vi "Modulacion FM.vi"() -> ()   [LabVIEW 2014]
doc: "This example demonstrates how to simulate a Frequency Modulation (FM) using the signal generation functions. This VI also presents the Power Spectrum of the FM signal."
uses:
  <vilib>/measure/maspectr.llb/FFT Power Spectrum and PSD for 1 Chan.vi
  <vilib>/measure/NI_MABase.lvlib
  <vilib>/measure/NI_MAPro.lvlib
panel:
  in  "Informacion de muestreo":cluster{"Fs":dbl, "#s":dbl}={"Fs"=4000000.0, "#s"=200.0} {"#s" format="%.2p"}
  in  "Frecuencia de Portadora":dbl(knob)=476774.62691567314 min=86453.20197044335 scale=62781.48791441017..1000000.0 scale format="%#_6p"
  in  "Desviacion de frecuencia\n(Maxima separacion entre\nla frecuencia modulada y\nla portadora).":dbl(slide)=35983.91523891873 scale=1.0..476774.62691567314 scale format="%#_6p"
  in  "Forma del del mensaje":T1(ring)=enum."Square Wave"
  in  "Frecuencia de mensaje":dbl(knob)=62781.48791441017 scale=1.0..100000.0 scale format="%#_6p"
  in  "Tab Control":T2(tab)=enum."Señal modulada y repsuesta en frecuencia"
  out "Mensaje":waveform(dbl)(graph)={"t0"=timestamp(0 s since 1904-01-01), "dt"=2.5e-07, "Y"=[1.0, 1.0, 1.0, 1.0, 1.0, 1.0, 1.0, 1.0, 1.0, 1.0, 1.0, 1.0, 1.0, 1.0, 1.0, 1.0, 1.0, 1.0, 1.0, 1.0, 1.0, 1.0, 1.0, 1.0, 1.0, 1.0, 1.0, 1.0, 1.0, 1.0, 1.0, 1.0, -1.0, -1.0, -1.0, -1.0, -1.0, -1.0, -1.0, -1.0, -1.0, -1.0, -1.0, -1.0, -1.0, -1.0, -1.0, -1.0, -1.0, -1.0, -1.0, -1.0, -1.0, -1.0, -1.0, -1.0, -1.0, -1.0, -1.0, -1.0, -1.0, -1.0, -1.0, -1.0, 1.0, 1.0, 1.0, 1.0, 1.0, 1.0, 1.0, 1.0, 1.0, 1.0, 1.0, 1.0, 1.0, 1.0, 1.0, 1.0, 1.0, 1.0, 1.0, 1.0, 1.0, 1.0, 1.0, 1.0, 1.0, 1.0, 1.0, 1.0, 1.0, 1.0, 1.0, 1.0, -1.0, -1.0, -1.0, -1.0, -1.0, -1.0, -1.0, -1.0, -1.0, -1.0, -1.0, -1.0, -1.0, -1.0, -1.0, -1.0, -1.0, -1.0, -1.0, -1.0, -1.0, -1.0, -1.0, -1.0, -1.0, -1.0, -1.0, -1.0, -1.0, -1.0, -1.0, -1.0, 1.0, 1.0, 1.0, 1.0, 1.0, 1.0, 1.0, 1.0, 1.0, 1.0, 1.0, 1.0, 1.0, 1.0, 1.0, 1.0, 1.0, 1.0, 1.0, 1.0, 1.0, 1.0, 1.0, 1.0, 1.0, 1.0, 1.0, 1.0, 1.0, 1.0, 1.0, 1.0, -1.0, -1.0, -1.0, -1.0, -1.0, -1.0, -1.0, -1.0, -1.0, -1.0, -1.0, -1.0, -1.0, -1.0, -1.0, -1.0, -1.0, -1.0, -1.0, -1.0, -1.0, -1.0, -1.0, -1.0, -1.0, -1.0, -1.0, -1.0, -1.0, -1.0, -1.0, -1.0, 1.0, 1.0, 1.0, 1.0, 1.0, 1.0, 1.0, 1.0]}
  out "Portadora":waveform(dbl)(graph)={"t0"=timestamp(0 s since 1904-01-01), "dt"=2.5e-07, "Y"=[0.0, 0.6808450864045564, 0.9973392598500482, 0.7801122137223073, 0.1454119376984075, -0.5671048245034954, -0.9761382177609353, -0.8627960252686081, -0.2877327661469225, 0.4413092733570824, 0.9341868169196235, 0.927138861399192, 0.42393708566906174, -0.3061325448566705, -0.872376843552464, -0.9717729476446748, -0.5511295189071326, 0.16444817223791786, 0.7920222295376438, 0.9957494703172831, 0.6666062596047739, -0.01926802565192162, -0.6948311213628872, -0.9985587460155945, -0.7679125490470704, -0.12632171297488315, 0.5828695690254743, 0.9801410562719645, 0.8528948583468899, 0.2692261547710468, -0.4585176067615233, -0.9408879170240065, -0.9197466673071168, -0.40640749383920877, 0.32441865922296087, 0.8816337559242037, 0.9670468667098986, 0.5349495837279978, -0.1834233486055864, -0.8036381744081004, -0.9937899676922854, -0.6521199277157222, 0.03852889725399705, 0.7085591715869883, 0.9994074760293471, 0.7554277651410067, 0.10718458610125767, -0.5984178991609463, -0.983779976958741, -0.8426770190042173, -0.25061958207241136, 0.4755556965783022, 0.9472396736523278, 0.9120129793005801, 0.3887270064520568, -0.3425843197710418, -0.8905633253730134, -0.9619617297092303, -0.5185710264348835, 0.20233042148395122, 0.8149557354346749, 0.9914614795212856, 0.6373914693860656, -0.05777546341261616, -0.7220241399715642, -0.9998851347652545, -0.7426624974954743, -0.08800766252580258, 0.6137440419505634, 0.9870536287217557, 0.8321463010352069, 0.2319199565091507, -0.4924172167132967, -0.9532397284527575, -0.9039406688304773, -0.3709021881183424, 0.3606227817496145, 0.8991622364276503, 0.9565194247096809, 0.5019999282432388, -0.22116237084178256, -0.8259707105056826, -0.9887648703516309, -0.622426353163902, 0.07700057804565562, 0.7352210270913103, 0.999991544872796, 0.7296214857429955, 0.06879806247295789, -0.6288423069311999, -0.9899607960826671, -0.8213066144035787, -0.21313422108911634, 0.5090959066311663, 0.9588858536572893, 0.8955327330752689, 0.352939657037624, -0.37852734763509865, -0.9074272963874506, -0.9507219723916216, -0.4852424418572703, 0.23991220454055817, 0.8366790098569661, 0.985701141410782, 0.6072301354663423, -0.09619710303575618, -0.7481449330571586, -0.9997266668428259, -0.7163095718974755, -0.04956291829965433, 0.6437070882487739, 0.9925003996355927, 0.8101619837904227, 0.1942693507919983, -0.525585573679836, -0.9641759529088857, -0.8867922938281574, -0.33484608254100134, 0.3962913696183658, 0.915355436507748, 0.9445715252985263, 0.4683047891854941, -0.25857296093058374, -0.847076657590386, -0.9822714302345698, -0.5918084585164578, 0.11535791088064368, 0.760791059335561, 0.9990905990222465, 0.7027316985564028, 0.030309371847132, -0.6583328667396499, -0.9946714964478871, -0.7987165470998694, -0.17533234997957645, 0.5418800953897728, 0.9691080620398415, 0.877722596337991, 0.31662818261485176, -0.41390825207301213, -0.9229437131392746, -0.9380703670377495, -0.4511932590305974, 0.27713771143579263, 0.8571597931500393, 0.978477010244836, 0.5761670482483742, -0.1344758873395082, -0.7731547105301447, -0.9980835775774913, -0.6888929070657068, -0.011044571789236884, 0.6727142119798575, 0.996473280410243, 0.786974553922721, 0.15633024979506188, -0.5579734217472057, -0.97368034980106, -0.8683270081043309, -0.29829272140650015, 0.4313714540042576, 0.9301893088211111, 0.9312209114326423, 0.43391420475446013, -0.29559956312626606, -0.86692467275565, -0.9743192902766233, -0.5603117121812814, 0.15354393407446035, 0.7852312961250714, 0.9967059764068381, 0.6747983356479502, -0.008224329021820102, -0.6868457843013597, -0.9979050825359921, -0.7749403639586171, -0.13727010555249414, 0.5738595774404425, 0.9778911185419804, 0.8586090176271293, 0.2798465067127493, -0.4486744914775589, -0.9370895333267855, -0.924025701626322, -0.41647404191920623, 0.3139516612775165, 0.8763676707926014, 0.9697998140550874, 0.5442483372631518, -0.17255497128608052, -0.7970163321894562, -0.9949583070015845, -0.6604532174945502, 0.02749017621125308, 0.7007223367746264, 0.998966371209495, 0.7626184453973145, 0.11815899411716616, -0.589532664078453, -0.9817388048409004]}
  out "Respuesta en frecuencia":cluster{"f0":dbl, "df":dbl, "magnitude":dbl[]}(graph)={"f0"=0.0, "df"=20000.0, "magnitude"=[2.88641475174006e-06, 1.030418592205968e-05, 1.25338793313667e-05, 1.5578991702681184e-06, 7.851169184240917e-06, 3.1038033624009525e-05, 1.315052190134009e-05, 7.136805871670306e-06, 3.772119577081144e-05, 1.8740446582511433e-05, 9.164661751380538e-06, 0.00014474065301626633, 9.329771771573295e-05, 2.001110050605276e-05, 0.00024055702815761184, 0.00025224842276803217, 2.7424587064414548e-05, 0.002025573217633073, 0.0022926865099421223, 0.0006854818461400615, 0.02906425333296893, 0.05075730279663054, 0.006914169119278008, 0.14348894661447417, 0.3665428704536463, 0.0543120641496029, 0.017556929983781368, 0.05647440941927177, 0.013067677987635681, 0.0005970530798616534, 0.003059081206333798, 0.000990649606028714, 4.959624687332605e-05, 0.00031000972296511435, 0.00015621110498333532, 8.340447202135528e-06, 0.00014818534888832858, 9.56659923019101e-05, 5.494888838215459e-06, 2.9801359805969647e-05, 3.046111398998357e-05, 2.7820099108281927e-07, 2.166646468729281e-05, 2.6814045321484444e-05, 2.795820636598245e-06, 4.992593291910251e-06, 1.0349397557477865e-05, 6.356985131000261e-07, 4.328162288378599e-06, 1.0383074708456256e-05, 2.147515532870235e-06, 1.0929487234750402e-06, 4.249400501587737e-06, 8.566560281440759e-07, 8.993800191361328e-07, 4.519361147047011e-06, 1.7612614153320688e-06, 3.917161491604026e-07, 1.85250448570518e-06, 8.62125474043589e-07, 1.508356279624567e-07, 2.0376378822576994e-06, 1.432489813952379e-06, 2.7881710497934736e-07, 8.282910690210554e-07, 7.652236770290614e-07, 1.3119040763240095e-08, 9.230167757288734e-07, 1.1224310788503782e-06, 2.7090968344331666e-07, 4.0347976209559703e-07, 6.261326725147224e-07, 2.3345456525957103e-08, 4.2042317106007244e-07, 8.376035654561846e-07, 2.8163623584234073e-07, 2.463793775724712e-07, 4.845570219999251e-07, 6.953811918423449e-08, 1.9532202113547189e-07, 5.992002839612192e-07, 2.952583130720333e-07, 1.963925397964037e-07, 3.7081362993089107e-07, 1.2067975869958115e-07, 9.1587895925322e-08, 4.2327452603486113e-07, 3.0248955357691745e-07, 1.7985998254704353e-07, 3.021148696115593e-07, 1.6552091093653498e-07, 4.092772617104061e-08, 3.1018745081273554e-07, 2.9723747901155125e-07, 1.7153366258991016e-07, 2.7822929908531567e-07, 2.0324040983178372e-07, 1.869047524872061e-08, 2.4457737435624293e-07, 2.837453893675089e-07]}
  out "Señal modulada":waveform(dbl)[](graph)=[{"t0"=timestamp(0 s since 1904-01-01), "dt"=2.5e-07, "Y"=[1.0, 1.0, 1.0, 1.0, 1.0, 1.0, 1.0, 1.0, 1.0, 1.0, 1.0, 1.0, 1.0, 1.0, 1.0, 1.0, 1.0, 1.0, 1.0, 1.0, 1.0, 1.0, 1.0, 1.0, 1.0, 1.0, 1.0, 1.0, 1.0, 1.0, 1.0, 1.0, -1.0, -1.0, -1.0, -1.0, -1.0, -1.0, -1.0, -1.0, -1.0, -1.0, -1.0, -1.0, -1.0, -1.0, -1.0, -1.0, -1.0, -1.0, -1.0, -1.0, -1.0, -1.0, -1.0, -1.0, -1.0, -1.0, -1.0, -1.0, -1.0, -1.0, -1.0, -1.0, 1.0, 1.0, 1.0, 1.0, 1.0, 1.0, 1.0, 1.0, 1.0, 1.0, 1.0, 1.0, 1.0, 1.0, 1.0, 1.0, 1.0, 1.0, 1.0, 1.0, 1.0, 1.0, 1.0, 1.0, 1.0, 1.0, 1.0, 1.0, 1.0, 1.0, 1.0, 1.0, -1.0, -1.0, -1.0, -1.0, -1.0, -1.0, -1.0, -1.0, -1.0, -1.0, -1.0, -1.0, -1.0, -1.0, -1.0, -1.0, -1.0, -1.0, -1.0, -1.0, -1.0, -1.0, -1.0, -1.0, -1.0, -1.0, -1.0, -1.0, -1.0, -1.0, -1.0, -1.0, 1.0, 1.0, 1.0, 1.0, 1.0, 1.0, 1.0, 1.0, 1.0, 1.0, 1.0, 1.0, 1.0, 1.0, 1.0, 1.0, 1.0, 1.0, 1.0, 1.0, 1.0, 1.0, 1.0, 1.0, 1.0, 1.0, 1.0, 1.0, 1.0, 1.0, 1.0, 1.0, -1.0, -1.0, -1.0, -1.0, -1.0, -1.0, -1.0, -1.0, -1.0, -1.0, -1.0, -1.0, -1.0, -1.0, -1.0, -1.0, -1.0, -1.0, -1.0, -1.0, -1.0, -1.0, -1.0, -1.0, -1.0, -1.0, -1.0, -1.0, -1.0, -1.0, -1.0, -1.0, 1.0, 1.0, 1.0, 1.0, 1.0, 1.0, 1.0, 1.0]}, {"t0"=timestamp(0 s since 1904-01-01), "dt"=2.5e-07, "Y"=[0.9984029777810175, 0.6509488431215257, -0.09645535030128369, -0.7845963259940434, -0.9906727738784062, -0.5880690799748571, 0.17585066138485858, 0.8317258411824421, 0.9765796057475771, 0.5214122245144965, -0.25411650621337517, -0.8735132879152705, -0.9562139920007735, -0.4514064051780484, 0.3307501932987203, 0.9096902707790675, 0.9297067383643397, 0.3785012603687799, -0.40525951429272977, -0.9400244296505748, -0.8972280975303089, -0.3031650504857898, 0.47716590537831616, 0.9643209321160209, 0.8589866756451884, 0.2258816503475007, -0.5460075210235095, -0.9824237248547382, -0.815228092459421, -0.1471474413257228, 0.6113422003561121, 0.9942165359496375, 0.8338275463663957, 0.2894125064540818, -0.38829381443560673, -0.8871682646648453, -0.9774501634232173, -0.6175594488052699, 0.02675328689073392, 0.6587445789708, 0.9873457036952253, 0.8612167435816471, 0.3384474158570927, -0.3401966187202963, -0.8621603368560242, -0.9870491078326964, -0.6573443936053383, -0.024894378767231495, 0.6190209444491316, 0.977841142895757, 0.8863086591937452, 0.3865795223038472, -0.2911919540786492, -0.8348526104243956, -0.9940151148617401, -0.6953758829673651, -0.07647563907626465, 0.5776460816643719, 0.9657282068119917, 0.9090363609274488, 0.43368043418620983, -0.24141053965353962, -0.8053179282843859, -0.9983296028003267, -0.649973402872853, 0.09773353470553524, 0.7853919241350666, 0.9904969615934172, 0.5870298782465428, -0.1771147556965716, -0.8324381547650586, -0.9763024853780582, -0.52031593596602, 0.25535839131683574, 0.8741377418406534, 0.9558373434553331, 0.45026007113022104, -0.33196189272511023, -0.9102228542597056, -0.9292329808083009, -0.37731224357823523, 0.4064332454519675, 0.9404617219710456, 0.8966602738477215, 0.3019409878549508, -0.4782941295456295, -0.9646601246038086, -0.8583284328947735, -0.2246304038737258, 0.5470829917597055, 0.9826626389199761, 0.814483658449982, 0.14587704760471293, -0.6123580100505189, -0.9943536370779119, -0.7654075598789647, -0.17832309303785954, 0.49088952296336175, 0.9340189812744355, 0.9469784099741436, 0.5237992388950001, -0.140619926898628, -0.7402754429906262, -0.9989910899620429, -0.7976132748454581, -0.2288881863463464, 0.4452532158169199, 0.9143296322866634, 0.9623041087737355, 0.567081610396859, -0.08931493050710693, -0.7045767545891988, -0.9953400305030686, -0.8276913694232525, -0.27884272415461586, 0.3984292029865556, 0.8922013239322462, 0.9750628770738914, 0.6088513009612416, -0.03777168799662689, -0.666998619197928, -0.9890339177627947, -0.8555616107861207, -0.32805345354863064, 0.35054238676203825, 0.867693083112449, 0.9852206810684722, 0.6489968906205055, -0.09901155791748559, -0.786186226926118, -0.9903195156779153, -0.5859897083275533, 0.17837855789222584, 0.8331490954041707, 0.9760237547890318, 0.5192187892584365, -0.2565998552567024, -0.8747607540472399, -0.9554591184436236, -0.44911299446669606, 0.33317304464545283, 0.9107539365062297, 0.9287576906646727, 0.37612260448513296, -0.40760630627926303, -0.9408974631843201, -0.8960909712998371, -0.3007164272316588, 0.47942156486056525, 0.9649977260738797, 0.8576687744999172, 0.22337878691614838, -0.5481575601897822, -0.9828999322758801, -0.8137378811094597, -0.1446064132881165, 0.6133728097804657, 0.9944890982148437, 0.7645804536250302, 0.06490525120522475, -0.5870755113863562, -0.9686738779236388, -0.9041416206682399, -0.4231995949464248, 0.2526504422177531, 0.8121402657363344, 0.9975922922031956, 0.7235950842534494, 0.11634028190746284, -0.54449598239644, -0.9545601986300204, -0.9249939607263338, -0.46941423974219054, 0.20235802278363701, 0.7809326539999161, 0.9998424072741465, 0.7582666173563534, 0.16746497680710182, -0.5004640192630023, -0.9379002455908458, -0.9433788944957768, -0.5143767297171693, 0.15152581662747228, 0.7476419171585739, 0.9994254590472672, 0.7909154866370308, 0.2181429616151649, -0.4550970765288298, -0.9187384589588549, -0.9592473804658946, -0.5579671281634178, 0.10028941782928638, 0.7869792330571499, 0.9901404364245631, 0.5849485719334467, -0.17964206588742654, -0.8338586619272212, -0.9757434144402092, -0.5181207862012718, 0.2578408959854246]}]
  in  "Stop":bool
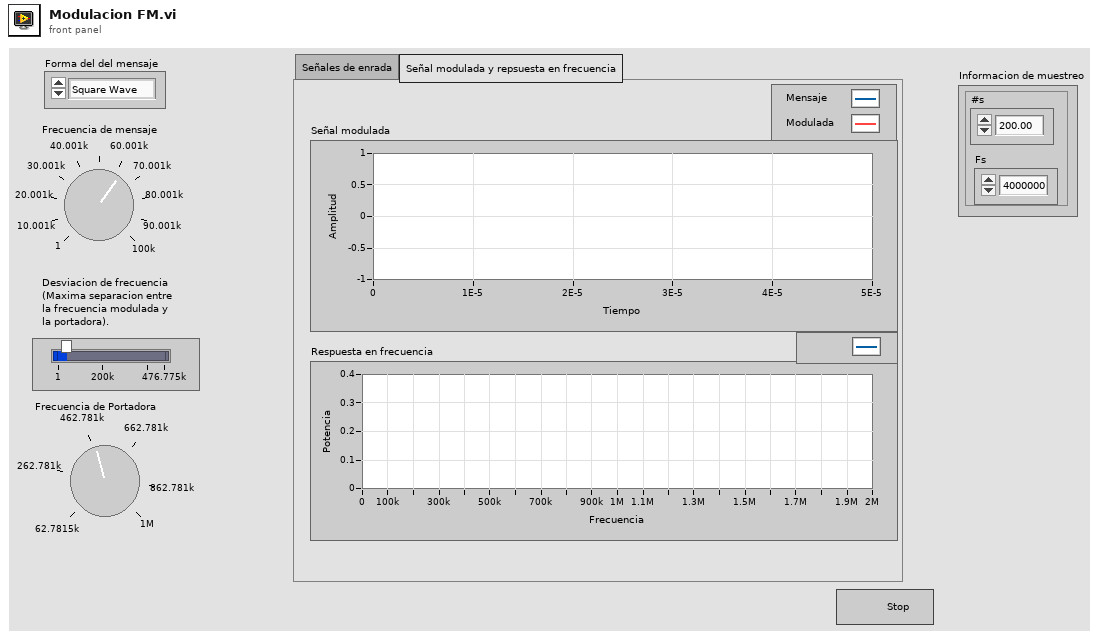
[diagram p1: front panel]
types:
  T1 = enum16{"Sine Wave", "Triangle Wave", "Square Wave", "Sawtooth Wave"}
  T2 = enum32{"Señales de enrada", "Señal modulada y repsuesta en frecuencia"}
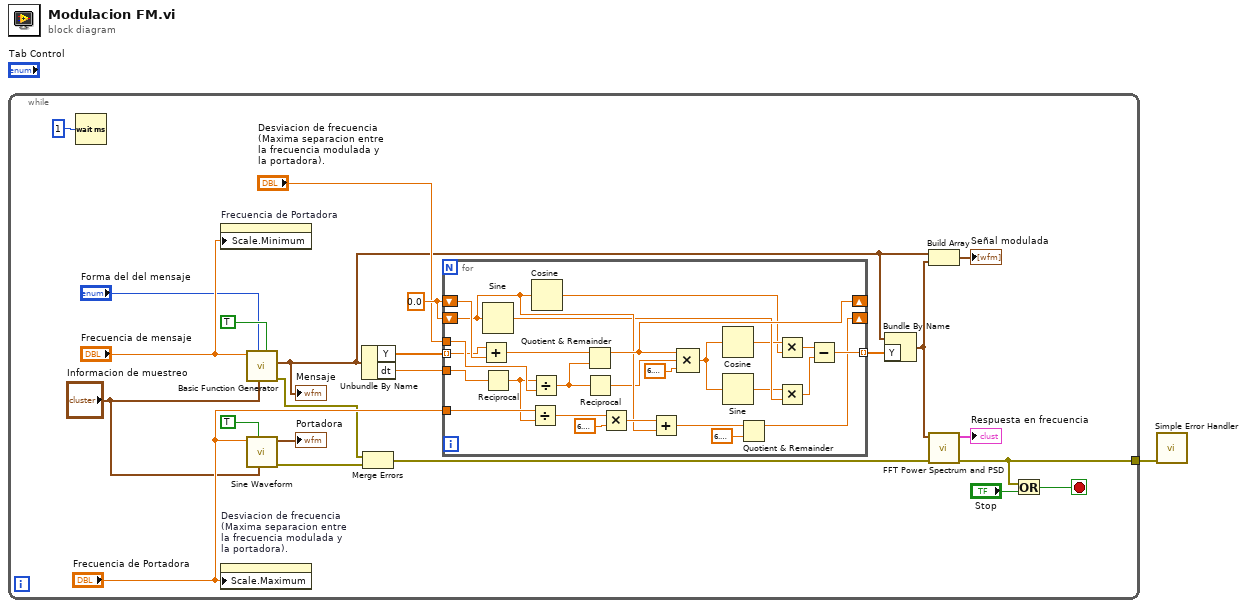
[diagram p0: block diagram]
diagram:
  n1 = while {
    tunnel: [w3] -> w1
    stop <- w4 stop-if-true
    w22 = 0.0
    n2 = Wait (ms)(milliseconds to wait=u32 1) -> ()  [unwired: 1 out]
    n3 = property on="Frecuencia de Portadora" class="Knob (strict)"("Scale.Minimum"="Frecuencia de mensaje") -> ()  [unwired: 2 in, 2 out]
    n4 = property on="Desviacion de frecuencia\n(Maxima separacion entre\nla frecuencia modulada y\nla portadora)." class="Slide (strict)"("Scale.Maximum"="Frecuencia de Portadora") -> ()  [unwired: 2 in, 2 out]
    n5 = call <vilib>:"Basic Function Generator.vi"("reset signal"=TRUE, "sampling info"="Informacion de muestreo", "signal type"="Forma del del mensaje", "frequency"="Frecuencia de mensaje") -> ("error out"=w6:errorcluster, "signal out"=w11:waveform(dbl))  [unwired: 5 in, 1 out]
    "Mensaje" <- w11
    n6 = call <vilib>:"Sine Waveform.vi"("sampling info"="Informacion de muestreo", "reset signal"=TRUE, "frequency"="Frecuencia de Portadora") -> ("error out"=w7:errorcluster, "signal out"=→"Portadora":waveform(dbl))  [unwired: 7 in]
    n7 = Unbundle By Name(w11) -> ("Y"=w16:dbl[], "dt"=w19:dbl)
    n8 = Merge Errors(w6, w7) -> (w5:errorcluster)
    n9 = for {
      tunnel: w19 -> [w50]
      tunnel: "Desviacion de frecuencia\n(Maxima separacion entre\nla frecuencia modulada y\nla portadora)." -> [w49]
      shift-right: [w36] -> _
      shift-left: w22 -> [w35]
      tunnel: w16 -> [w34] mode=indexing
      tunnel: "Frecuencia de Portadora" -> [w48]
      tunnel: [w43] -> w18 mode=indexing
      shift-right: [w39] -> _
      shift-left: w22 -> [w32]
      n10 = Add(x=w34, y=w35) -> (x+y=w38:dbl)
      n11 = Sine(x=w32) -> (sin(x)=w31:dbl)
      n12 = Reciprocal(x=w50) -> (1/x=w47:dbl)
      n13 = Divide(x=w48, y=w47) -> (x/y=w45:dbl)
      n14 = Divide(x=w47, y=w49) -> (x/y=w37:dbl)
      n15 = Cosine(x=w32) -> (cos(x)=w29:dbl)
      n16 = Quotient & Remainder(x=w38, y=w37) -> (x-y*floor(x/y)=w36:dbl)  [unwired: 1 out]
      n17 = Reciprocal(x=w37) -> (1/x=w26:dbl)
      n18 = Multiply(x=w45, y=6.283185307179586) -> (x*y=w42:dbl)
      n19 = Add(x=w42, y=w32) -> (x+y=w41:dbl)
      n20 = Compound Arithmetic op=MULTIPLY(w36, w26, 6.283185307179586) -> (w27:dbl)
      n21 = Cosine(x=w27) -> (cos(x)=w30:dbl)
      n22 = Sine(x=w27) -> (sin(x)=w28:dbl)
      n23 = Quotient & Remainder(x=w41, y=6.283185307179586) -> (x-y*floor(x/y)=w39:dbl)  [unwired: 1 out]
      n24 = Multiply(x=w30, y=w29) -> (x*y=w44:dbl)
      n25 = Multiply(x=w28, y=w31) -> (x*y=w33:dbl)
      n26 = Subtract(x=w44, y=w33) -> (x-y=w43:dbl)
    }
    n27 = Bundle By Name(cluster=w11, "Y"=w18) -> (w9:waveform(dbl))
    n28 = Build Array(w11, w9) -> (→"Señal modulada":waveform(dbl)[])
    n29 = call-poly <vilib>:"FFT Power Spectrum and PSD.vi"("error in (no error)"=w5, "time signal"=w9) -> ("error out"=w3:errorcluster, "Power Spectrum / PSD"=→"Respuesta en frecuencia":cluster{"f0":dbl, "df":dbl, "magnitude":dbl[]})  [unwired: 6 in, 2 out]
    n30 = Or(x=w3, y="Stop") -> (x .or. y?=w4:bool)
  }
  n31 = call <vilib>:"Simple Error Handler.vi"("error in (no error)"=w1) -> ()  [unwired: 4 in, 5 out]
